vi "Error Handler - CMH.vi"(11 "error in (no error)":errorcluster) -> (3 "error dup":errorcluster, 5 "channel":T1)   [LabVIEW 2023]
uses:
  <extravilib>/ChannelInstances/Messenger-t'Message Queue.lvlib-Message Cluster.ctl'/))Channel.ctl
  Message Cluster.ctl
  <extravilib>/ChannelInstances/Messenger-t'Message Queue.lvlib-Message Cluster.ctl'/Write.vi
  <extravilib>/ChannelInstances/Messenger-t'Message Queue.lvlib-Message Cluster.ctl'/Write With Abort.vi
  <extravilib>/ChannelInstances/Messenger-t'Message Queue.lvlib-Message Cluster.ctl'/Endpoint.vi
  Message Queue.lvlib
  <extravilib>/ChannelInstances/Messenger-t'Message Queue.lvlib-Message Cluster.ctl'.lvlib
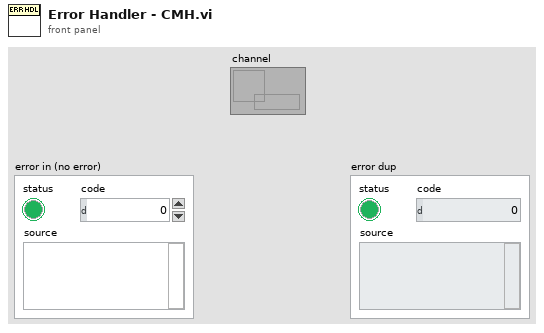
[diagram p1: front panel]
types:
  T1 = typedef "Messenger-t'Message Queue.lvlib-Message Cluster.ctl'.lvlib/))Channel.ctl" = refnum<queue>
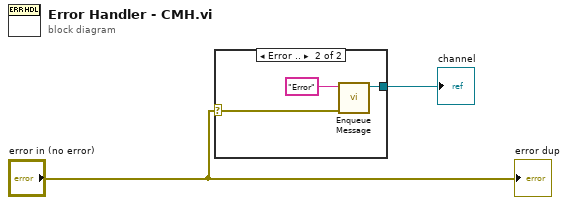
[diagram p0: block diagram]
diagram:
  n1 = case shown="Error .." "error in (no error)" {
    selector: "error in (no error)" -> [_ w4]
    tunnel: [_ w3] -> w1
    frame No Error {
    }
    frame Error {
      n2 = call "Enqueue Message.vi"("Message Data"=w4, "Message"="Error") -> ("channel"=w3:T1)  [unwired: 9 in]
    }
  }
  "channel" <- w1
  "error dup" <- "error in (no error)"
